vi "StoreAccno.vi"(7 "Enum":enum16{"Read", "Write"}(ring)=enum."Write", 11 "Numeric":i32) -> (3 "Read":i32)   [LabVIEW 2017]
doc: "This VI has the information about the current account number."
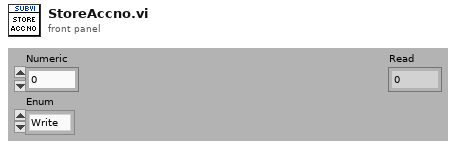
[diagram p1: front panel]
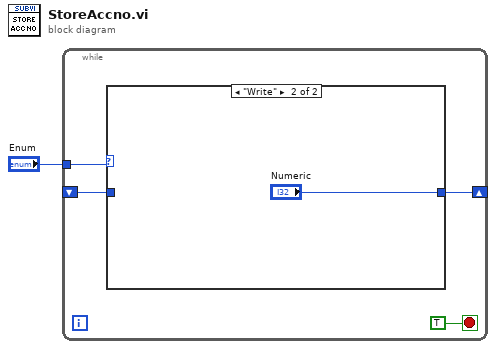
[diagram p0: block diagram]
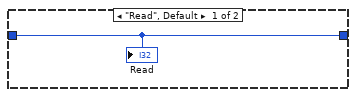
[diagram p2: hidden frame]
diagram:
  n1 = while {
    shift-right: [w5] -> _
    shift-left: _ -> [w4]
    tunnel: "Enum" -> [w3]
    stop <- TRUE stop-if-true
    n2 = case shown="\"Write\"" w3 {
      tunnel: [w6 "Numeric"] -> w5
      tunnel: w4 -> [w6 _]
      frame "Read", Default {
        "Read" <- w6
      }
      frame "Write" {
      }
    }
  }
